vi "Extract_multipart_message.vi"(0 "multipart message in":string[](array[string]), 11 "error in (no error)":errorcluster) -> (3 "Valid message?":bool, 4 "command out":T2=enum."configure_rf", 6 "parameters":string, 8 "datatype":T1, 10 "data out":string, 13 "datatype":string, 14 "Debug info":string, 15 "error out":errorcluster)   [LabVIEW 2019, in "mmW_commands.lvlib"]
uses:
  mmW_commands.lvlib
  TypeDefs/commands.ctl
  commands/typedefs/datatypes_.ctl
panel:
  out "command_prefix":string
  out "command":string
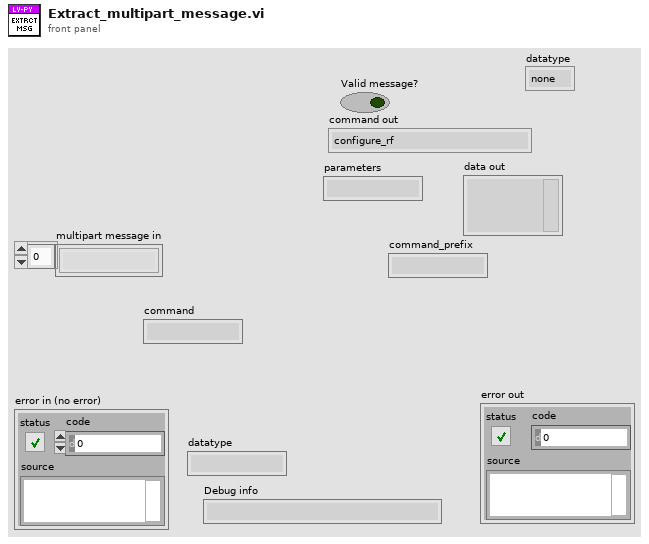
[diagram p1: front panel]
types:
  T1 = typedef "mmW_commands.lvlib/datatypes_.ctl" = enum16{"none", "string", "interleaved_I16", "interleaved_I32", "I16_array", "I32_array", "JSONstring"}
  T2 = typedef "mmW_commands.lvlib/commands.ctl" = enum16{"configure_fs", "configure_rf", "configure_trigger", "equalization_enable", "equalization_start", "lo_sync_enable", "equalization_stop", "get_instrument_status", "get_versions", "initialize_hw", "pop_rx", "set_log_level", "Shutdown", "start", "start_instrument_app", "stop", "trans", "transceive", "trigger_burst", "trigger_sync_enable", "Write TX", "resp_generic", "resp_waveform", "send_trigger", "fetch", "transceive2"}
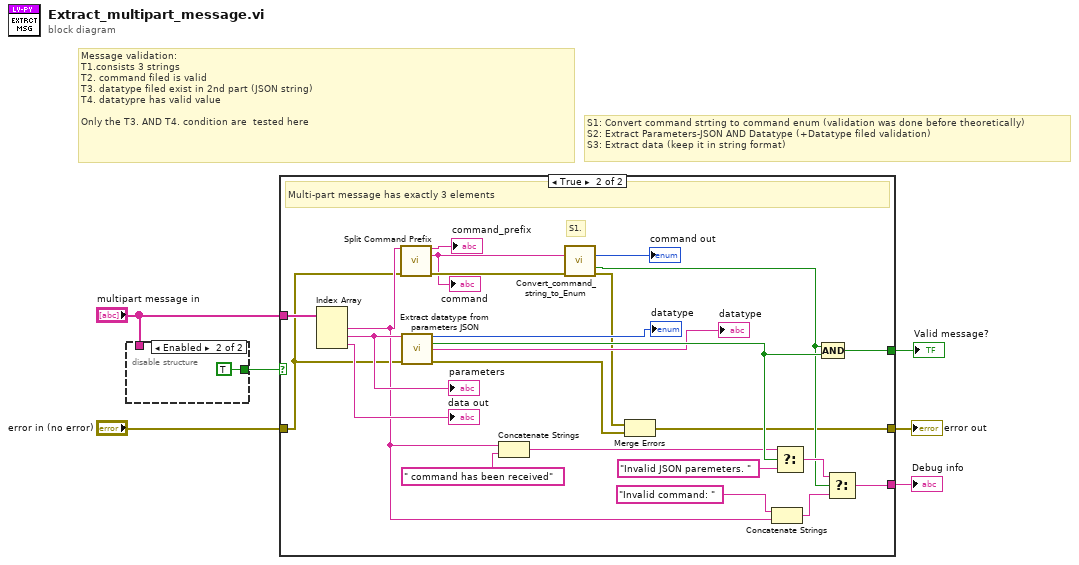
[diagram p0: block diagram]
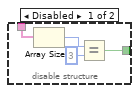
[diagram p2: hidden frame]
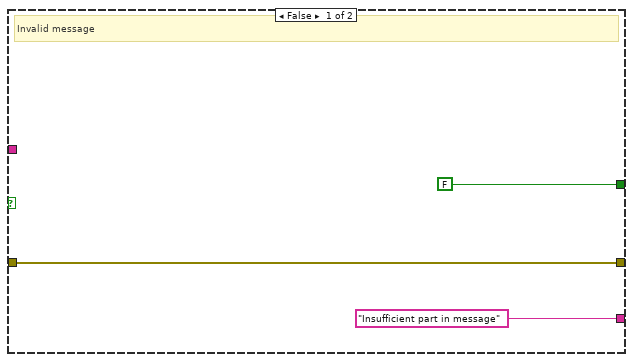
[diagram p3: hidden frame]
diagram:
  # "S1: Convert command strting to command enum (validation was done before theoretically)\nS2: Extract Parameters-JSON AND Datatype (+Datatype filed validation)\nS3: Extract data (keep it in string format)"
  # "Message validation:\nT1.consists 3 strings\nT2. command filed is valid\nT3. datatype filed exist in 2nd part (JSON string)\nT4. datatypre has valid value\n\nOnly the T3. AND T4. condition are  tested here"
  n1 = disable-structure shown="Enabled" {
    disable-tunnel: "multipart message in" -> [w10 _]
    disable-tunnel: [w9 TRUE] -> w4
    frame Disabled {
      n2 = Array Size(array=w10) -> (size(s)=w7:i32)
      n3 = Equal?(x=w7, y=3) -> (x = y?=w9:bool)
    }
    frame Enabled {
    }
  }
  n4 = case shown="True" w4 {
    tunnel: "error in (no error)" -> [w13 w20]
    tunnel: "multipart message in" -> [_ w38]
    tunnel: [FALSE w34] -> w2
    tunnel: [w13 w16] -> w1
    tunnel: ["Insufficient part in message" w27] -> w6
    frame False {
      # "Invalid message"
    }
    frame True {
      # "S1."
      # "Multi-part message has exactly 3 elements"
      n5 = Index Array(array=w38) -> (element #1=w22:string, element #2=w36:string, element #3=→"data out":string)  [unwired: 3 in]
      "parameters" <- w36
      n6 = call "Split Command Prefix.vi"("command string in"=w22, "error in"=w20) -> ("command prefix"=→"command_prefix":string, "command out"=w15:string, "error out"=w19:errorcluster)  [unwired: 11 in]
      "command" <- w15
      n7 = call "Extract datatype from parameters JSON.vi"("parameters JSON in"=w36, "error in (no error)"=w20) -> ("datatype enum"=→"datatype":T1, "datatype valid?"=w33:bool, "datatype string"=→"datatype":string, "error out"=w17:errorcluster)  [unwired: 10 in]
      n8 = Concatenate Strings(w22, " command has been received" ("string")) -> (w32:string)
      n9 = call "Convert_command_string_to_Enum.vi"("Command field in"=w15, "error in (no error)"=w19) -> ("mmW_instrument_commands"=→"command out":T2, "Found in Enum?"=w25:bool, "error out"=w18:errorcluster)  [unwired: 11 in]
      n10 = Merge Errors(w18, w17) -> (w16:errorcluster)
      n11 = Concatenate Strings("Invalid command: " ("f"), w22) -> (w28:string)
      n12 = Select(t=w32, s=w33, f="Invalid JSON paremeters. ") -> (s? t:f=w30:string)
      n13 = Compound Arithmetic op=AND(w25, w33) -> (w34:bool)
      n14 = Select(t=w30, s=w25, f=w28) -> (s? t:f=w27:string)
    }
  }
  "Debug info" <- w6
  "error out" <- w1
  "Valid message?" <- w2
